vi "Load Pictures.vi"(10 "Application Directory":path) -> (1 "Map":picture, 2 "Vortex":picture, 3 "Mars":picture)   [LabVIEW 2019, in "LSS.lvlib"]
doc: "Loads a set of images that are used in the front panel of the example."
uses:
  LSS.lvlib
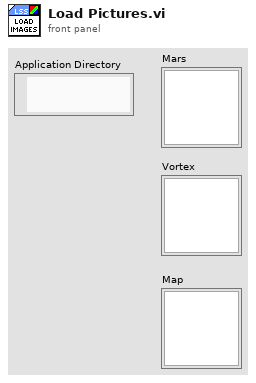
[diagram p1: front panel]
types:
  T1 = typedef "imagedata.ctl" = cluster{"image type":i32, "image depth":i32, "image":u8[], "mask":u8[], "colors":u32[], "Rectangle":cluster{"left":i16, "top":i16, "right":i16, "bottom":i16}}
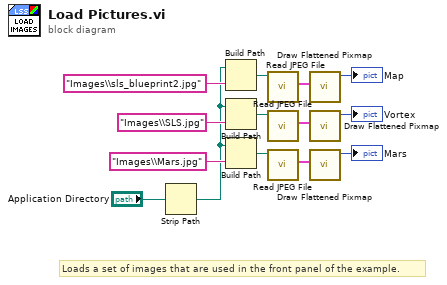
[diagram p0: block diagram]
diagram:
  # "Loads a set of images that are used in the front panel of the example."
  n1 = Strip Path(path="Application Directory") -> (stripped path=w1:path)  [unwired: 1 out]
  n2 = Build Path(base path=w1, name or relative path="Images\\sls_blueprint2.jpg") -> (appended path=w3:path)
  n3 = Build Path(base path=w1, name or relative path="Images\\SLS.jpg") -> (appended path=w4:path)
  n4 = Build Path(base path=w1, name or relative path="Images\\Mars.jpg") -> (appended path=w7:path)
  n5 = call <vilib>:"Read JPEG File.vi"("path to JPEG file"=w3) -> ("image data"=w11:T1)  [unwired: 8 in, 2 out]
  n6 = call <vilib>:"Read JPEG File.vi"("path to JPEG file"=w4) -> ("image data"=w12:T1)  [unwired: 8 in, 2 out]
  n7 = call <vilib>:"Read JPEG File.vi"("path to JPEG file"=w7) -> ("image data"=w13:T1)  [unwired: 8 in, 2 out]
  n8 = call <vilib>:"Draw Flattened Pixmap.vi"("image data"=w11) -> ("new picture"=→"Map":picture)  [unwired: 8 in]
  n9 = call <vilib>:"Draw Flattened Pixmap.vi"("image data"=w12) -> ("new picture"=→"Vortex":picture)  [unwired: 8 in]
  n10 = call <vilib>:"Draw Flattened Pixmap.vi"("image data"=w13) -> ("new picture"=→"Mars":picture)  [unwired: 8 in]
